vi "Sequence.Test.Print.vi"(7 "Code in":T1={"Ready"=FALSE, "DoubleOrder"=FALSE, "OrderDone"=FALSE, "AllowSingleSlot"=FALSE, "CheckDM"=FALSE, "ThresholdA"=0, "ThresholdB"=0, "Plate"=enum."Wabco", "ImgPath"=path "", "Variant"={"State"=enum."Init", "ImgPath"=path "", "WabcoPlate"="", "WabcoProduct"="", "ClientProduct"="", "ClientPlate"="", "TotalQuantity"=0, "OrderQuantity"=0, "Serial"=0, "Wabco"={"LaserJob"="", "AdditionalTxt"="037", "FactoryCode"="", "RevID"=0, "ForkID"=0, "FailuresLimit"=0, "GlobalCnt"=0, "Bank"=0, "SerialFormat"=enum."6 dig", "CoordA"={"X"=0.0, "Y"=0.0, "Angle"=0.0}, "CoordB"={"X"=0.0, "Y"=0.0, "Angle"=0.0}, "DMCconfig"=0}, "Client"={"LaserJob"="", "AdditionalTxt"="", "FactoryCode"="037", "RevID"=0, "ForkID"=0, "FailuresLimit"=0, "GlobalCnt"=0, "Bank"=0, "SerialFormat"=enum."6 dig", "CoordA"={"X"=0.0, "Y"=0.0, "Angle"=0.0}, "CoordB"={"X"=0.0, "Y"=0.0, "Angle"=0.0}, "DMCconfig"=0}}}, 8 "error in":errorcluster, 11 "Data in":T8) -> (0 "error out":errorcluster, 3 "Data out":T8)   [LabVIEW 2016]
uses:
  Sequence.Test.Status.ctl
  Sequence.Slot.StatusData.ctl
  Sequence.Test.Unload.Status.ctl
  Sequence.Prod.StatusData.ctl
  Sequence.Step.Status.ctl
  Sequence.Test.BreakReason.ctl
  Sequence.Code.Sets.ctl
  Sequence.PlateType.ctl
  Logger/Logger.Variant.Sets.ctl
  Station/Station.Changeover.State.vi
  Station/Station.Plate.Properties.ctl
  Sequence.Code.SerialFormat.ctl
  Drivers/V7310/LowLevel/V7310.Job.Sets.ctl
  Station/Station.ProductSlot.ctl
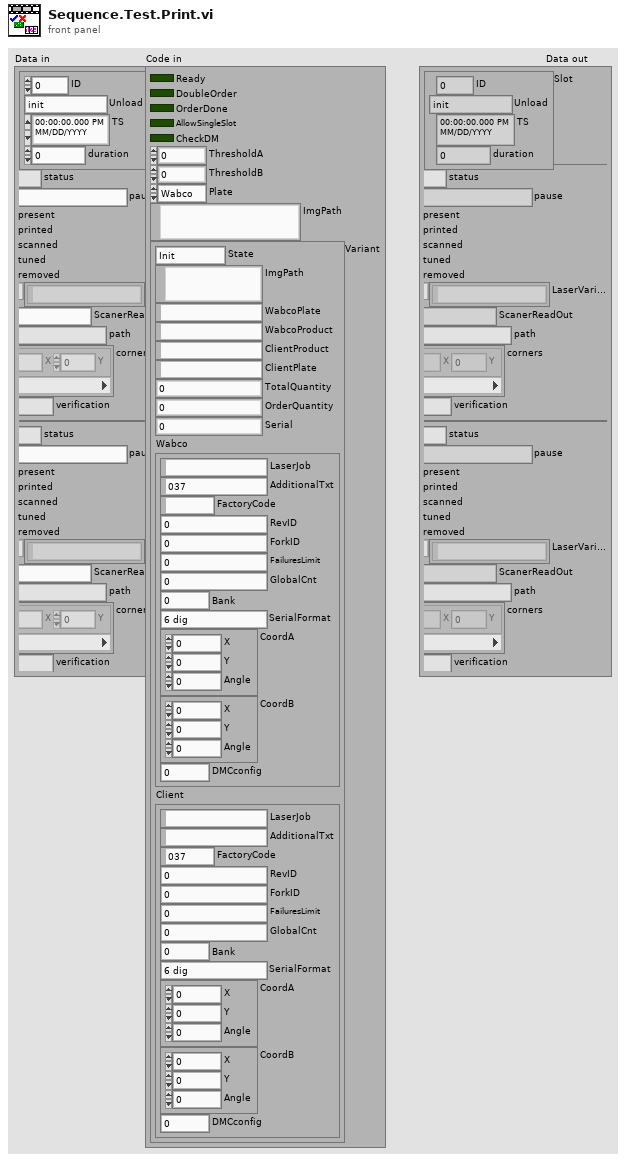
[diagram p1: front panel]
types:
  T1 = typedef "Sequence.Code.Sets.ctl" = cluster{"Ready":bool, "DoubleOrder":bool, "OrderDone":bool, "AllowSingleSlot":bool, "CheckDM":bool, "ThresholdA":u8, "ThresholdB":u8, "Plate":T2, "ImgPath":path, "Variant":T3}
  T2 = typedef "Sequence.PlateType.ctl" = enum16{"Wabco", "Client"}
  T3 = typedef "Logger.Variant.Sets.ctl" = cluster{"State":T4, "ImgPath":path, "WabcoPlate":string, "WabcoProduct":string, "ClientProduct":string, "ClientPlate":string, "TotalQuantity":u16, "OrderQuantity":u16, "Serial":i32, "Wabco":T5, "Client":T5}
  T4 = typedef "Station.Changeover.State.vi" = enum16{"Init", "Scaning", "NOK", "Wait for ack", "Ready"}
  T5 = typedef "Station.Plate.Properties.ctl" = cluster{"LaserJob":string, "AdditionalTxt":string, "FactoryCode":string, "RevID":u8, "ForkID":u8, "FailuresLimit":u16, "GlobalCnt":i32, "Bank":u8, "SerialFormat":T6, "CoordA":T7, "CoordB":T7, "DMCconfig":i32}
  T6 = typedef "Sequence.Code.SerialFormat.ctl" = enum8{"", "6 dig", "7 dig"}
  T7 = typedef "V7310.Job.Sets.ctl" = cluster{"X":dbl, "Y":dbl, "Angle":dbl}
  T8 = typedef "Sequence.Test.Status.ctl" = cluster{"Slot":T9, "A":T11, "B":T11}
  T9 = typedef "Sequence.Slot.StatusData.ctl" = cluster{"ID":i32, "Unload":T10, "TS":timestamp, "duration":u32}
  T10 = typedef "Sequence.Test.Unload.Status.ctl" = enum16{"init", "check NOK", "check OK", "wait on NOK", "wait on OK", "wait on Unload", "done"}
  T11 = typedef "Sequence.Prod.StatusData.ctl" = cluster{"status":T12, "pause":T13, "present":bool, "printed":bool, "scanned":bool, "tuned":bool, "removed":bool, "LaserVariables":string[], "ScanerReadOut":string, "path":path, "corners":cluster{"X":i32, "Y":i32}[], "verification":u8}
  T12 = typedef "Sequence.Step.Status.ctl" = enum16{"-", "Pending", "Running", "Skipped", "Passed", "Failed", "Done", "Error", "Aborted", "Stopped"}
  T13 = typedef "Sequence.Test.BreakReason.ctl" = enum16{"-", "NOK container", "OK container", "Rev empty", "Rev missing", "Rev wrong", "Fork missing", "Fork wrong", "NOK limit", "Unload failure", "Single slot", "Part done", "Err: Prod move work", "Err: Prod move home", "Err: Prod lift work", "Err: Prod lift home", "Err: Prod Arm Work", "Err: Prod Arm NOK", "Err: Prod Arm OK", "Err: Prod NOK suck", "Err: Prod NOK drop", "Err: Prod OK missing", "Err: Prod OK suck", "Err: Prod OK drop"}
  T14 = typedef "Station.ProductSlot.ctl" = enum8{"A", "B"}
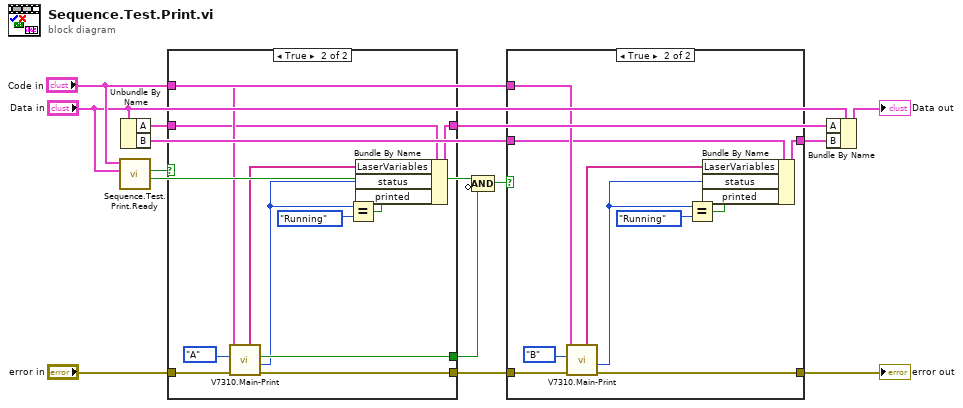
[diagram p0: block diagram]
diagram:
  n1 = call "Sequence.Test.Print.Ready.vi"("Data in"="Data in", "Code in"="Code in") -> ("Print B"=w9:bool, "Print A"=w13:bool)  [unwired: 8 in]
  n2 = Unbundle By Name("Data in") -> ("A"=w11:T11, "B"=w7:T11)
  n3 = case shown="True" w13 {
    tunnel: "error in" -> [w16 w23]
    tunnel: [w16 w24] -> w8
    tunnel: "Code in" -> [_ w26]
    tunnel: [_ w27] -> w12
    tunnel: w11 -> [w15 w18]
    tunnel: [w15 w17] -> w3
    frame False {
    }
    frame True {
      n4 = call "V7310.Main-Print.vi"("error in"=w23, "Slot"=Station.ProductSlot."A", "Code sets in"=w26) -> ("error out"=w24:errorcluster, "Status"=w21:T12, "Aborted"=w27:bool, "LaserVars"=w22:string[])  [unwired: 4 in, 1 out]
      n5 = Equal?(x=w21, y=Sequence.Step.Status."Running") -> (x = y?=w19:bool)
      n6 = Bundle By Name(cluster=w18, "LaserVariables"=w22, "status"=w21, "printed"=w19) -> (w17:T11)
    }
  }
  n7 = Compound Arithmetic op=AND(w9, invert w12) -> (w10:bool)
  n8 = case shown="True" w10 {
    tunnel: w8 -> [w29 w36]
    tunnel: [w29 w37] -> w1
    tunnel: "Code in" -> [_ w39]
    tunnel: w7 -> [w28 w31]
    tunnel: [w28 w30] -> w2
    frame False {
    }
    frame True {
      n9 = call "V7310.Main-Print.vi"("error in"=w36, "Slot"=Station.ProductSlot."B", "Code sets in"=w39) -> ("error out"=w37:errorcluster, "Status"=w34:T12, "LaserVars"=w35:string[])  [unwired: 4 in, 2 out]
      n10 = Equal?(x=w34, y=Sequence.Step.Status."Running") -> (x = y?=w32:bool)
      n11 = Bundle By Name(cluster=w31, "LaserVariables"=w35, "status"=w34, "printed"=w32) -> (w30:T11)
    }
  }
  "error out" <- w1
  n12 = Bundle By Name(cluster="Data in", "A"=w3, "B"=w2) -> (→"Data out":T8)
